vi "Curtin1_NewWAVTest.vi"(11 "Settings":T1={"Name of test"="", "Date"=timestamp(0 s since 1904-01-01), "Location"="", "Template"="", "Soundcard"="", "resolution"=32, "Sampling rate"=48000, "Ch1 Gain "=25.0, "Ch2 Gain"=10.0, "Sample time (s)"=0.3, "Pre-trigger (s)"=0.01, "Hammer Threshold"=10.0, "Positions"=12, "Taps/Position"=5, "Set Names"="", "Freq resolution"=10.0, "Hammer cutoff"=0.0, "Mic cutoff"=0.0, "Double bounce "=0.0, "Hammer Cal"=1.0, "dB Offset"=0.0, "Accel Cal"=1.0, "Vibrometer Cal"=1.0, "Mic Cal"=1.0, "Output"=2, "Voltage Cal"=1.0, "Vibrometer Port"="ASRL27::INSTR", "Range"=50, "High Pass"=2, "Bandwidth"=25, "X Range"=[], "Y Range"=[], "dB Spread"=0.0, "Trigger"=0, "Ch_1"=1, "Ch_2"=2, "flip?"=FALSE, "60Hz"=FALSE, "Time offset"=0.0, "Piezo Cal"=1.0, "Default Notes"=""} {"Ch_2" min=1 step=1; "Ch_1" min=1 max=100 step=1; "Trigger" items=["Hammer (force)", "Self-tap", "Spacebar"]; "Bandwidth" items=["1 kHz"=1, "5 kHz"=5, "10 kHz"=10, "25 kHz"=25, "50 kHz"=50, "100 kHz"=100]; "High Pass" items=["Off", "13 Hz", "104 Hz"]; "Range" items=["10 mm/s"=1, "20 mm/s"=2, "50 mm/s"=5, "100 mm/s"=10, "200 mm/s"=20, "500 mm/s"=50, "1 m/s"=100, "2 m/s"=200]; "Output" items=["Accelerometer", "Speed (from acceleration)", "Microphone", "Vibrometer", "Piezo"]; "Voltage Cal" format="%#_13g"; "Ch2 Gain" format="%#_13g"; "Ch1 Gain" format="%#_13g"; "Double bounce" min=0.0; "Mic cutoff" min=0.0 format="%#_4g"; "Hammer cutoff" min=0.0 format="%#_4g"; "Freq resolution" min=0.0; "Pre-trigger (s)" format="%#_13g"; "Date" format="%<%H:%M\n%d/%m/%y>T"; "resolution" items=["16 bit"=16, "24 bit"=24, "32 bit"=32]; "Sampling rate" items=["22050 samp/s"=22050, "44100 samp/s"=44100, "48000 samp/s"=48000]}) -> (0 "Instrument -- test out":string, 1 "updated?":bool, 3 "Settings out":T1={"Name of test"="", "Date"=timestamp(0 s since 1904-01-01), "Location"="", "Template"="", "Soundcard"="", "resolution"=32, "Sampling rate"=48000, "Ch1 Gain "=25.0, "Ch2 Gain"=10.0, "Sample time (s)"=0.3, "Pre-trigger (s)"=0.01, "Hammer Threshold"=10.0, "Positions"=12, "Taps/Position"=5, "Set Names"="", "Freq resolution"=10.0, "Hammer cutoff"=0.0, "Mic cutoff"=0.0, "Double bounce "=0.0, "Hammer Cal"=1.0, "dB Offset"=0.0, "Accel Cal"=1.0, "Vibrometer Cal"=1.0, "Mic Cal"=1.0, "Output"=2, "Voltage Cal"=1.0, "Vibrometer Port"="ASRL27::INSTR", "Range"=50, "High Pass"=2, "Bandwidth"=25, "X Range"=[], "Y Range"=[], "dB Spread"=0.0, "Trigger"=0, "Ch_1"=1, "Ch_2"=2, "flip?"=FALSE, "60Hz"=FALSE, "Time offset"=0.0, "Piezo Cal"=1.0, "Default Notes"=""} {"Ch_2" min=1 step=1; "Ch_1" min=1 max=100 step=1; "Trigger" items=["Hammer (force)", "Self-tap", "Spacebar"]; "Bandwidth" items=["1 kHz"=1, "5 kHz"=5, "10 kHz"=10, "25 kHz"=25, "50 kHz"=50, "100 kHz"=100]; "High Pass" items=["Off", "13 Hz", "104 Hz"]; "Range" items=["10 mm/s"=1, "20 mm/s"=2, "50 mm/s"=5, "100 mm/s"=10, "200 mm/s"=20, "500 mm/s"=50, "1 m/s"=100, "2 m/s"=200]; "Output" items=["Accelerometer", "Speed (from acceleration)", "Microphone", "Vibrometer", "Piezo"]; "Voltage Cal" format="%#_13g"; "Ch2 Gain" format="%#_13g"; "Ch1 Gain" format="%#_13g"; "Double bounce" min=0.0; "Mic cutoff" min=0.0 format="%#_4g"; "Hammer cutoff" min=0.0 format="%#_4g"; "Freq resolution" min=0.0; "Pre-trigger (s)" format="%#_13g"; "Date" format="%<%H:%M\n%d/%m/%y>T"; "resolution" items=["16 bit"=16, "24 bit"=24, "32 bit"=32]; "Sampling rate" items=["22050 samp/s"=22050, "44100 samp/s"=44100, "48000 samp/s"=48000]})   [LabVIEW 2022 SP3]
uses:
  PreferencesControl.ctl
  <vilib>/Utility/miscctls.llb/LVSelectionTypeDef.ctl
  <vilib>/Utility/error.llb/Trim Whitespace One-Sided.vi
panel:
  in  "OK Button":bool
  in  "Cancel Button":bool
  in  "Instrument Notes":string
  in  "Tag List":bool
  in  "Instrument Name":string(combo)
  in  "Instrument Keywords":string
  out "File name":string
  in  "Test Name":string
  # "New Test"
  # "Hz"
  # "dB"
  # "dB"
  # "sec"
  # "sec"
  # "mV/Pa"
  # "mV/m/s2"
  # "mV/mm/s"
  # "V/N"
  # "sec"
  # "sec"
  # "mV/N"
  # "a.u."
  # "a.u."
  # "sec"
  # "Hz"
  # "dB"
  # "dB"
  # "sec"
  # "sec"
  # "mV/Pa"
  # "mV/m/s2"
  # "mV/mm/s"
  # "V/N"
  # "sec"
  # "sec"
  # "mV/N"
  # "a.u."
  # "a.u."
  # "sec"
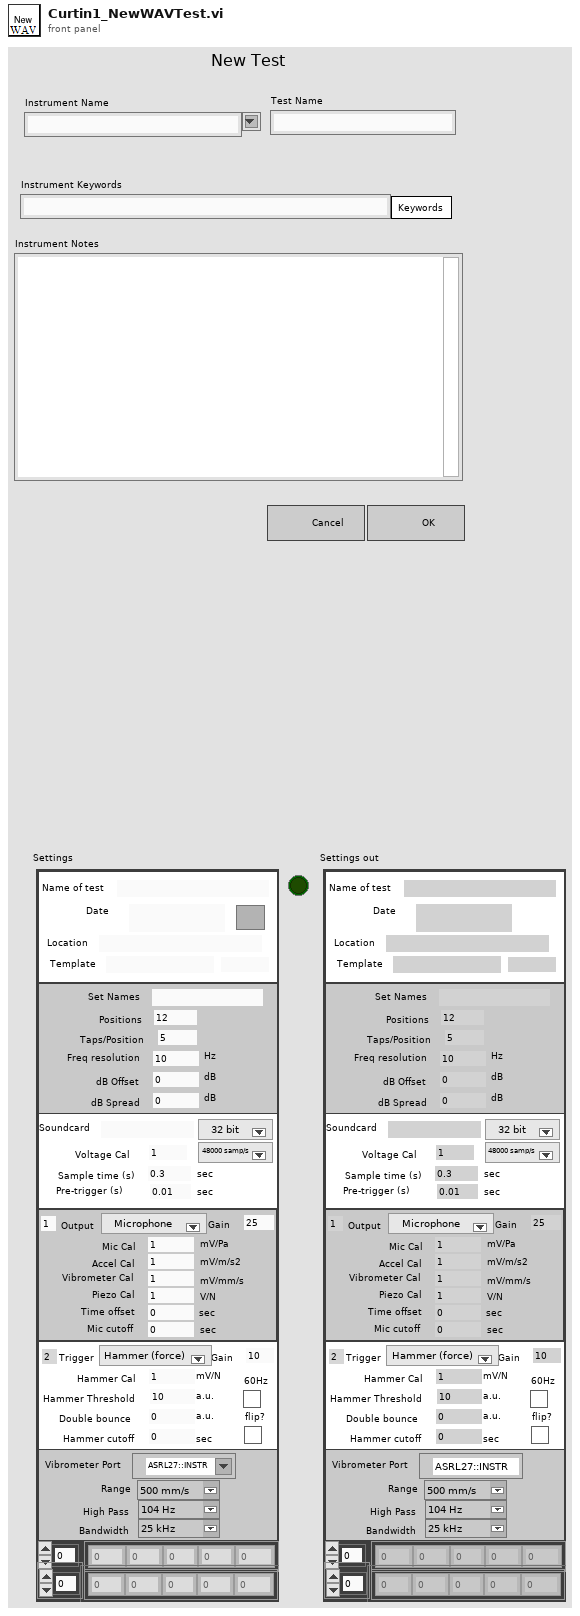
[diagram p1: front panel]
types:
  T1 = typedef "PreferencesControl.ctl" = cluster{"Name of test":string, "Date":timestamp, "Location":string, "Template":string, "Soundcard":string, "resolution":u16, "Sampling rate":u16, "Ch1 Gain ":dbl, "Ch2 Gain":dbl, "Sample time (s)":dbl, "Pre-trigger (s)":dbl, "Hammer Threshold":dbl, "Positions":i16, "Taps/Position":i16, "Set Names":string, "Freq resolution":dbl, "Hammer cutoff":dbl, "Mic cutoff":dbl, "Double bounce ":dbl, "Hammer Cal":dbl, "dB Offset":dbl, "Accel Cal":dbl, "Vibrometer Cal":dbl, "Mic Cal":dbl, "Output":u16, "Voltage Cal":dbl, "Vibrometer Port":refnum<visa-resource-name>, "Range":u16, "High Pass":u16, "Bandwidth":u16, "X Range":cluster{"Minimum":dbl, "Maximum":dbl, "Increment":dbl, "Minor Increment":dbl, "Start":dbl}[], "Y Range":cluster{"Minimum":dbl, "Maximum":dbl, "Increment":dbl, "Minor Increment":dbl, "Start":dbl}[], "dB Spread":dbl, "Trigger":u16, "Ch_1":u8, "Ch_2":u8, "flip?":bool, "60Hz":bool, "Time offset":dbl, "Piezo Cal":dbl, "Default Notes":string}
  T2 = enum8{"Enabled", "Disabled", "Disabled and Grayed Out"}
  T3 = typedef "LVSelectionTypeDef.ctl" = cluster{"Selection Start":u32, "Selection End":u32}
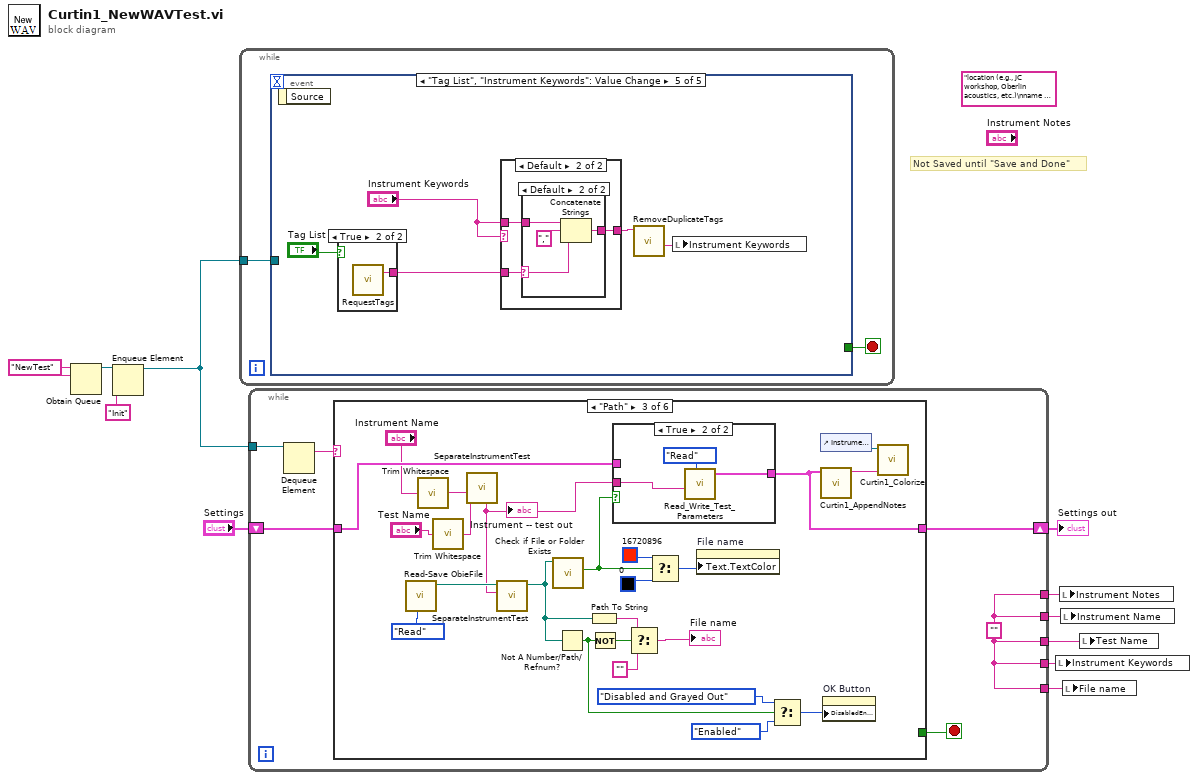
[diagram p0: block diagram]
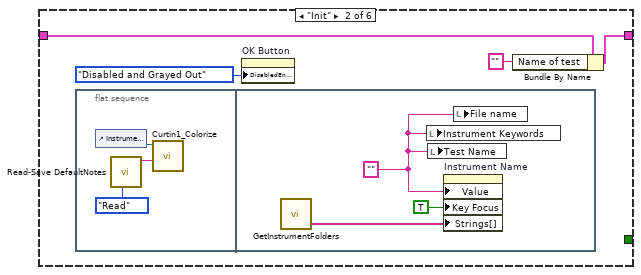
[diagram p3: hidden frame]
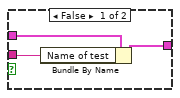
[diagram p4: hidden frame]
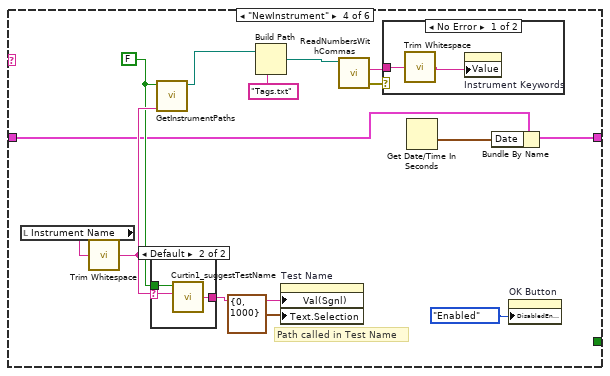
[diagram p5: hidden frame]
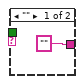
[diagram p7: hidden frame]
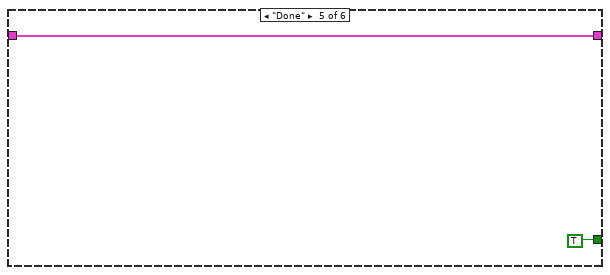
[diagram p8: hidden frame]
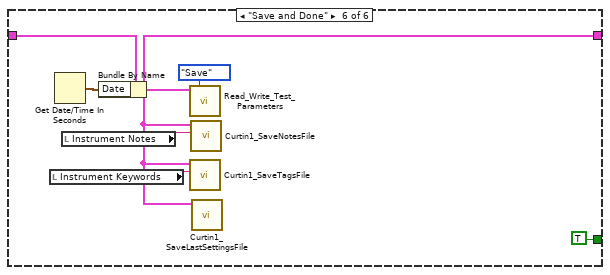
[diagram p9: hidden frame]
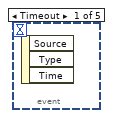
[diagram p10: hidden frame]
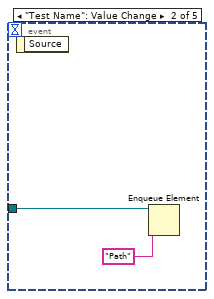
[diagram p11: hidden frame]
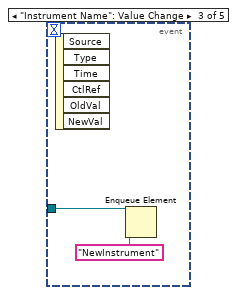
[diagram p12: hidden frame]
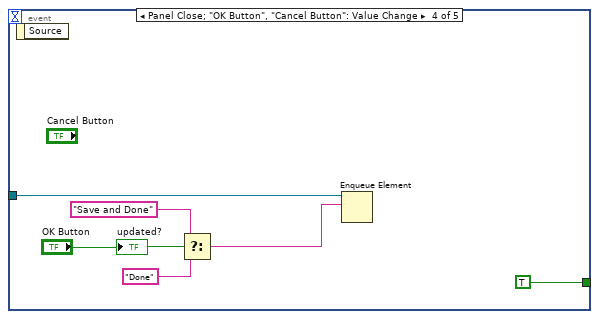
[diagram p13: hidden frame]
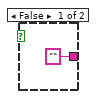
[diagram p16: hidden frame]
diagram:
  (unwired) "location (e.g., JC workshop, Oberlin acoustics, etc.)\nname of experiment (if applicable) \nnames of researchers\n\nInstrument Information:\ninstrument (e.g., violin, viola, cello, guitar, mandolin, etc.) \nmodel (e.g., Titian Strad, Guadagnini, personal, etc.) \nmaker name\nmaker ID (e.g., serial number)\nyear built (4 digits)\ncountry of origin \nsession (e.g. Oberlin 2017, VSA 2008) \nmaking school (e.g. Old Italian) \n\nMeasurement Information:\ntype (Radiation, admittance, modal analysis, taptones, etc.) \nprotocol (HV24, etc.)\n" ("Notes")
  w11 = "NewTest" ("name (unnamed)")
  # "Not Saved until \"Save and Done\""
  n1 = Obtain Queue(name (unnamed)=w11, element data type=w11) -> (queue out=w10:refnum<queue>)  [unwired: 3 in, 2 out]
  n2 = Enqueue Element(queue=w10, element="Init") -> (queue out=w8:refnum<queue>)  [unwired: 2 in, 2 out]
  n3 = while {
    tunnel: w8 -> [w12]
    stop <- w13 stop-if-true
    n4 = event shown="[4] \"Tag List\", \"Instrument Keywords\": Value Change" {
      selector: _ -> [_ _ _ _ _]
      dyn-events: _ -> [_ _ _ _ _]
      timeout: _ -> [_ _ _ _ _]
      tunnel: [_ _ _ TRUE _] -> w13
      tunnel: w12 -> [_ w14 w16 w22 _]
      event Timeout {
        n5 = event-data() -> ()  [unwired: 1 in, 3 out]
      }
      event "Test Name": Value Change {
        n6 = event-data() -> ()  [unwired: 1 in, 1 out]
        n7 = Enqueue Element(queue=w14, element="Path") -> ()  [unwired: 2 in, 3 out]
      }
      event "Instrument Name": Value Change {
        n8 = event-data() -> ()  [unwired: 1 in, 6 out]
        n9 = Enqueue Element(queue=w16, element="NewInstrument") -> ()  [unwired: 2 in, 3 out]
      }
      event Panel Close; "OK Button", "Cancel Button": Value Change {
        n10 = event-data() -> ()  [unwired: 1 in, 1 out]
        n11 = Select(t="Save and Done" ("element"), s="OK Button", f="Done" ("element")) -> (s? t:f=w19:string)
        n12 = Enqueue Element(queue=w22, element=w19) -> ()  [unwired: 2 in, 3 out]
        "updated?" <- "OK Button"
      }
      event "Tag List", "Instrument Keywords": Value Change {
        n13 = event-data() -> ()  [unwired: 1 in, 1 out]
        n14 = case shown="True" "Tag List" {
          tunnel: ["" ("Tags out") w39] -> w28
          frame False {
          }
          frame True {
            n15 = call "RequestTags.vi"() -> ("Tags out"=w39:string)  [unwired: 11 in]
          }
        }
        n16 = case shown="Default" "Instrument Keywords" {
          tunnel: w28 -> [w29 w30]
          tunnel: "Instrument Keywords" -> [_ w32]
          tunnel: [w29 w31] -> w26
          frame "" {
          }
          frame Default {
            n17 = case shown="Default" w30 {
              selector: w30 -> [_ w34]
              tunnel: w32 -> [w33 w37]
              tunnel: [w33 w36] -> w31
              frame "" {
              }
              frame Default {
                n18 = Concatenate Strings(w37, "," ("string"), w34) -> (w36:string)
              }
            }
          }
        }
        n19 = call "RemoveDuplicateTags.vi"("Tags"=w26) -> ("Tag string"=w24:string)  [unwired: 9 in, 1 out]
        n20 = local write "Instrument Keywords"(w24) -> ()
      }
    }
  }
  n21 = while {
    tunnel: w8 -> [w44]
    shift-right: [w41] -> w1
    shift-left: "Settings" -> [w42]
    tunnel: [w40] -> w7
    tunnel: [w40] -> w6
    tunnel: [w40] -> w5
    tunnel: [w40] -> w4
    tunnel: [w40] -> w3
    stop <- w43 stop-if-true
    w40 = "" ("Value (Signaling)")
    n22 = Dequeue Element(queue=w44) -> (element=w45:string)  [unwired: 2 in, 3 out]
    n23 = case shown="\"Path\"" w45 {
      tunnel: [_ _ _ _ TRUE TRUE] -> w43
      tunnel: w42 -> [w46 w47 w64 w90 w107 w110]
      tunnel: [w46 w49 w61 w94 w107 w109] -> w41
      frame Default {
      }
      frame "Init" {
        n24 = flat-sequence {
          frame #0 {
            n25 = control-ref of="Instrument Notes"() -> (w52:refnum<vi>)
            n26 = call "Read-Save DefaultNotes.vi"("Task"=enum16{"Save", "Read"}."Read") -> ("Notes Out"=w51:string)  [unwired: 9 in, 1 out]
            n27 = call "Curtin1_Colorize.vi"("Instrument Notes"=w51, "Text"=w52) -> ()  [unwired: 10 in]
          }
          frame #1 {
            w54 = "" ("Value (Signaling)")
            n28 = call "GetInstrumentFolders.vi"() -> ("folder names"=w56:string[])  [unwired: 11 in]
            n29 = local write "Instrument Keywords"(w54) -> ()
            n30 = local write "Test Name"(w54) -> ()
            n31 = property on="Instrument Name" class="CmbBox"("Value"=w54, "Key Focus"=TRUE, "Strings[]"=w56) -> ()  [unwired: 2 in, 2 out]
            n32 = local write "File name"(w54) -> ()
          }
        }
        n33 = property on="OK Button" class="Bool"("DisabledEnum"=T2."Disabled and Grayed Out" ("Disabled")) -> ()  [unwired: 2 in, 2 out]
        n34 = Bundle By Name(cluster=w47, "Name of test"="") -> (w49:T1)
      }
      frame "Path" {
        n35 = call "Read-Save ObieFile.vi"("Task"=enum16{"Save", "Read"}."Read") -> ("DataPath Out"=w67:path)  [unwired: 8 in, 2 out]
        n36 = call <vilib>:"Trim Whitespace.vi"("string"="Instrument Name") -> ("trimmed string"=w60:string)  [unwired: 1 in]
        n37 = call <vilib>:"Trim Whitespace.vi"("string"="Test Name") -> ("trimmed string"=w57:string)  [unwired: 1 in]
        n38 = call "SeparateInstrumentTest.vi"("test in"=w57, "Instrument in"=w60) -> ("Instrument -- test out"=w65:string)  [unwired: 5 in, 4 out]
        "Instrument -- test out" <- w65
        n39 = call "SeparateInstrumentTest.vi"("Instrument"=w65, "path in"=w67) -> ("path out"=w66:path)  [unwired: 5 in, 4 out]
        n40 = call <vilib>:"Check if File or Folder Exists.vi"("path"=w66) -> ("file or folder exists?"=w69:bool)  [unwired: 8 in, 2 out]
        n41 = Not A Number/Path/Refnum?(number/path/refnum=w66) -> (NaN/Path/Refnum?=w79:bool)
        n42 = Path To String(path=w66) -> (string=w78:string)
        n43 = Not(x=w79) -> (.not. x?=w77:bool)
        n44 = case shown="True" w69 {
          tunnel: w64 -> [w83 _]
          tunnel: [w82 w84] -> w61
          tunnel: w65 -> [w81 w85]
          frame False {
            n45 = Bundle By Name(cluster=w83, "Name of test"=w81) -> (w82:T1)
          }
          frame True {
            n46 = call "Read_Write_Test_Parameters.vi"("Task"=enum16{"Save", "Read", "Clear"}."Read", "Instrument Name"=w85) -> ("Settings"=w84:T1)  [unwired: 8 in, 1 out]
          }
        }
        n47 = Select(t=w78, s=w77, f="") -> (s? t:f=→"File name":string)
        n48 = Select(t=u32 16720896, s=w69, f=u32 0) -> (s? t:f=w76:u32)
        n49 = property on="File name" class="Str"("Text.TextColor"=w76) -> ()  [unwired: 2 in, 2 out]
        n50 = Select(t=T2."Disabled and Grayed Out" ("Disabled"), s=w79, f=T2."Enabled" ("Disabled")) -> (s? t:f=w80:T2)
        n51 = control-ref of="Instrument Notes"() -> (w63:refnum<vi>)
        n52 = call "Curtin1_AppendNotes.vi"("Settings"=w61) -> ("Instrument Notes"=w62:string)  [unwired: 10 in]
        n53 = property on="OK Button" class="Bool"("DisabledEnum"=w80) -> ()  [unwired: 2 in, 2 out]
        n54 = call "Curtin1_Colorize.vi"("Instrument Notes"=w62, "Text"=w63) -> ()  [unwired: 10 in]
      }
      frame "NewInstrument" {
        w93 = FALSE ("Build?")
        # "Path called in Test Name"
        n55 = local read "Instrument Name"() -> (w97:string)
        n56 = call <vilib>:"Trim Whitespace.vi"("string"=w97) -> ("trimmed string"=w95:string)  [unwired: 1 in]
        n57 = case shown="Default" w95 {
          selector: w95 -> [_ w106]
          tunnel: ["" w105] -> w100
          tunnel: w93 -> [_ w104]
          frame "" {
          }
          frame Default {
            n58 = call "Curtin1_suggestTestName.vi"("instrument"=w106, "Build?"=w104) -> ("Suggested Test"=w105:string)  [unwired: 9 in]
          }
        }
        n59 = call "GetInstrumentPaths.vi"("Instrument"=w95, "Build?"=w93) -> ("Path To Instrument Folder"=w96:path)  [unwired: 5 in, 4 out]
        n60 = Build Path(base path=w96, name or relative path="Tags.txt") -> (appended path=w87:path)
        n61 = property on="Test Name" class="Str"("Val(Sgnl)"=w100, "Text.Selection"=T3 {"Selection Start"=0, "Selection End"=1000}) -> ()  [unwired: 2 in, 2 out]
        n62 = call "ReadNumbersWithCommas.vi"("file (use dialog)"=w87) -> ("error out"=w89:errorcluster, "text"=w88:string)  [unwired: 7 in, 2 out]
        n63 = case shown="No Error" w89 {
          tunnel: w88 -> [w102 _]
          frame No Error {
            n64 = call <vilib>:"Trim Whitespace.vi"("string"=w102) -> ("trimmed string"=w101:string)  [unwired: 1 in]
            n65 = property on="Instrument Keywords" class="Str"("Value"=w101) -> ()  [unwired: 2 in, 2 out]
          }
          frame Error {
          }
        }
        n66 = Get Date/Time In Seconds() -> (seconds since 1Jan1904=w91:timestamp)
        n67 = Bundle By Name(cluster=w90, "Date"=w91) -> (w94:T1)
        n68 = property on="OK Button" class="Bool"("DisabledEnum"=T2."Enabled" ("Disabled")) -> ()  [unwired: 2 in, 2 out]
      }
      frame "Done" {
      }
      frame "Save and Done" {
        n69 = local read "Instrument Keywords"() -> (w111:string)
        n70 = Get Date/Time In Seconds() -> (seconds since 1Jan1904=w114:timestamp)
        n71 = local read "Instrument Notes"() -> (w112:string)
        n72 = Bundle By Name(cluster=w110, "Date"=w114) -> (w109:T1)
        n73 = call "Read_Write_Test_Parameters.vi"("Task"=enum16{"Save", "Read", "Clear"}."Save", "Settings"=w109) -> ()  [unwired: 8 in, 2 out]
        n74 = call "Curtin1_SaveTagsFile.vi"("Tags"=w111, "Settings in"=w109) -> ()  [unwired: 10 in]
        n75 = call "Curtin1_SaveNotesFile.vi"("Notes"=w112, "Settings in"=w109) -> ()  [unwired: 10 in]
        n76 = call "Curtin1_SaveLastSettingsFile.vi"("Settings in"=w109) -> ()  [unwired: 11 in]
      }
    }
  }
  "Settings out" <- w1
  n77 = local write "Instrument Keywords"(w4) -> ()
  n78 = local write "Instrument Notes"(w7) -> ()
  n79 = local write "Instrument Name"(w6) -> ()
  n80 = local write "File name"(w3) -> ()
  n81 = local write "Test Name"(w5) -> ()
